vi "Add Channel.vi"(8 "error in (no error)":errorcluster, 11 "Parent Ref in":T3 format="%.0x") -> (0 "error out":errorcluster, 1 "Cancelled?":bool, 2 "Channel Settings":T2, 3 "Parent Ref out":T3 format="%.0x")   [LabVIEW 2011, in "Ethernet IP Custom Device Custom Device.lvlib"]
uses:
  Ethernet IP Custom Device Custom Device.lvlib
  L5K Data Types.ctl
  <vilib>/NI Veristand/Custom Device API/Custom Device Item Ref.ctl
  <vilib>/NI Veristand/Custom Device API/Custom Device API.lvlib
panel:
  in  "Same":bool=TRUE
  in  "Tag Name":string
  in  "Cancel":bool
  in  "OK":bool
  in  "Data Type":T1=enum."REAL"
  in  "Number of Elements":u16=1 min=1 max=256
  in  "Channel Name":string
  # "Please enter the following channel settings:"
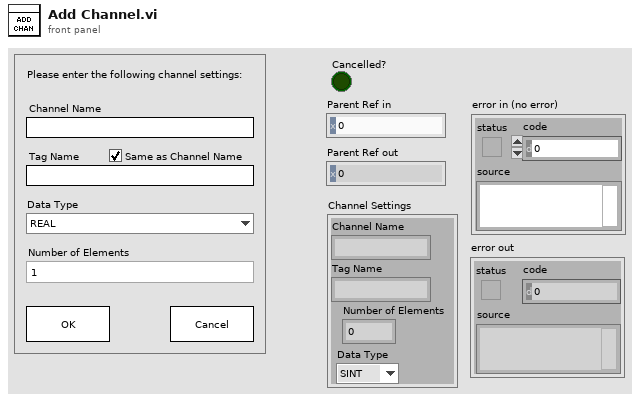
[diagram p1: front panel]
types:
  T1 = typedef "Ethernet IP Custom Device Custom Device.lvlib/L5K Data Types.ctl" = enum16{"SINT", "INT", "DINT", "REAL", "BOOL"}
  T2 = cluster{"Channel Name":string, "Tag Name":string, "Number of Elements":u16, "Data Type":T1}
  T3 = typedef "Custom Device API.lvlib/Custom Device Item Ref.ctl" = u64
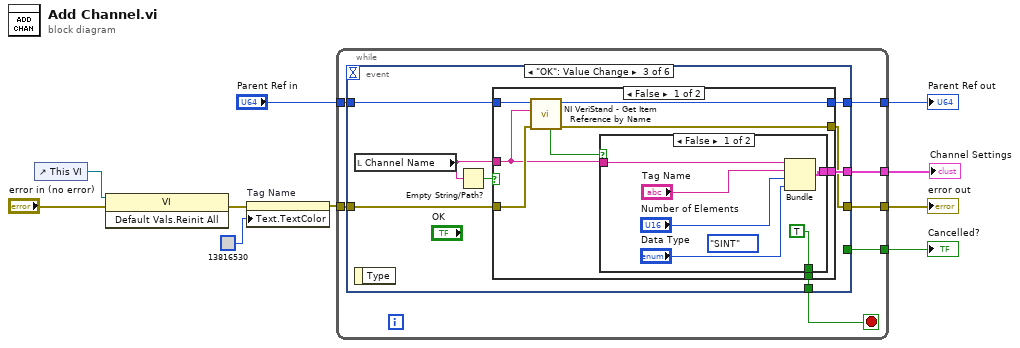
[diagram p0: block diagram]
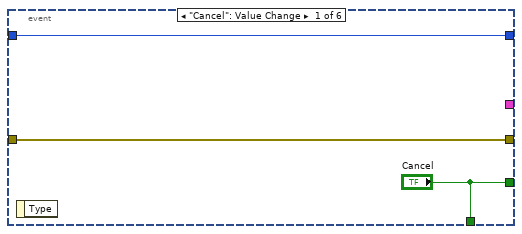
[diagram p2: hidden frame]
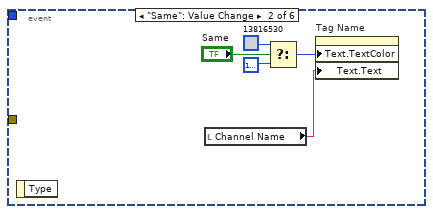
[diagram p3: hidden frame]
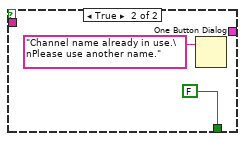
[diagram p4: hidden frame]
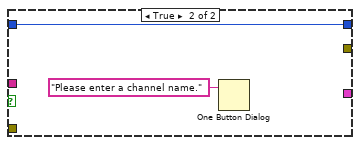
[diagram p5: hidden frame]
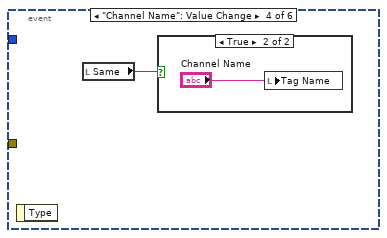
[diagram p6: hidden frame]
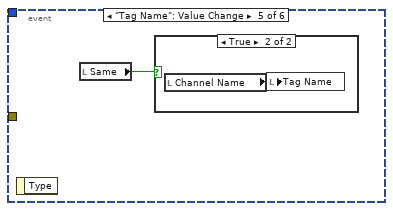
[diagram p8: hidden frame]
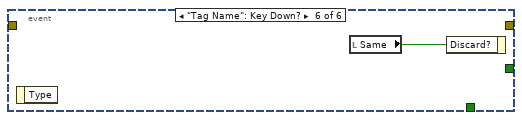
[diagram p10: hidden frame]
diagram:
  n1 = control-ref of="This VI"() -> (w6:refnum<vi>)
  n2 = invoke class="VI" method="Default Vals.Reinit All"(reference=w6, error in="error in (no error)") -> (error out=w4:errorcluster)  [unwired: 1 in, 2 out]
  n3 = property on="Tag Name" class="Str"(error in=w4, "Text.TextColor"=u32 13816530) -> (error out=w3:errorcluster)  [unwired: 1 in, 1 out]
  n4 = while {
    tunnel: "Parent Ref in" -> [w17]
    tunnel: [w15] -> w9
    tunnel: w3 -> [w14]
    tunnel: [w13] -> w1
    tunnel: [w12] -> w8
    tunnel: [w11] -> w7
    stop <- w16 stop-if-true
    n5 = event shown="[2] \"OK\": Value Change" {
      selector: _ -> [_ _ _ _ _ _]
      dyn-events: _ -> [_ _ _ _ _ _]
      timeout: _ -> [_ _ _ _ _ _]
      tunnel: w17 -> [w19 _ w33 _ _ _]
      tunnel: ["Cancel" _ w30 _ _ _] -> w16
      tunnel: ["Cancel" _ _ _ _ _] -> w15
      tunnel: w14 -> [w18 _ w32 _ _ _]
      tunnel: [_ _ w31 _ _ _] -> w13
      tunnel: [w19 _ w29 _ _ _] -> w12
      tunnel: [w18 _ w28 _ _ _] -> w11
      event "Cancel": Value Change {
        n6 = event-data() -> ()  [unwired: 1 in, 1 out]
      }
      event "Same": Value Change {
        n7 = event-data() -> ()  [unwired: 1 in, 1 out]
        n8 = local read "Channel Name"() -> (w22:string)
        n9 = Select(t=u32 13816530, s="Same", f=u32 16777228) -> (s? t:f=w25:u32)
        n10 = property on="Tag Name" class="Str"("Text.TextColor"=w25, "Text.Text"=w22) -> ()  [unwired: 2 in, 2 out]
      }
      event "OK": Value Change {
        n11 = local read "Channel Name"() -> (w26:string)
        n12 = event-data() -> ()  [unwired: 1 in, 1 out]
        n13 = Empty String/Path?(string/path=w26) -> (empty?=w27:bool)
        n14 = case shown="False" w27 {
          tunnel: w33 -> [w41 w50]
          tunnel: w32 -> [w40 _]
          tunnel: w26 -> [w38 _]
          tunnel: [w37 _] -> w31
          tunnel: [w36 _] -> w30
          tunnel: [w35 w50] -> w29
          tunnel: [w34 _] -> w28
          frame False {
            n15 = call <vilib>:"NI VeriStand - Get Item Reference by Name.vi"("error in (no error)"=w40, "Item Name"=w38, "Parent Ref in"=w41) -> ("error out"=w34:errorcluster, "Parent Ref out"=w35:T3, "Found"=w39:bool)  [unwired: 5 in, 1 out]
            n16 = case shown="False" w39 {
              tunnel: w38 -> [w43 _]
              tunnel: [w45 _] -> w37
              tunnel: [TRUE FALSE] -> w36
              frame False {
                (unwired) L5K_Data_Types."SINT" ("Data Type")
                n17 = Bundle("Channel Name"=w43, "Tag Name"="Tag Name", "Number of Elements"="Number of Elements", "Data Type"="Data Type") -> (w45:T2)  [unwired: 1 in]
              }
              frame True {
                n18 = One Button Dialog(message="Channel name already in use.\nPlease use another name.") -> ()  [unwired: 1 in, 1 out]
              }
            }
          }
          frame True {
            n19 = One Button Dialog(message="Please enter a channel name.") -> ()  [unwired: 1 in, 1 out]
          }
        }
      }
      event "Channel Name": Value Change {
        n20 = event-data() -> ()  [unwired: 1 in, 1 out]
        n21 = local read "Same"() -> (w52:bool)
        n22 = case shown="True" w52 {
          frame False {
          }
          frame True {
            n23 = local write "Tag Name"("Channel Name") -> ()
          }
        }
      }
      event "Tag Name": Value Change {
        n24 = event-data() -> ()  [unwired: 1 in, 1 out]
        n25 = local read "Same"() -> (w54:bool)
        n26 = case shown="True" w54 {
          frame False {
          }
          frame True {
            n27 = local read "Channel Name"() -> (w55:string)
            n28 = local write "Tag Name"(w55) -> ()
          }
        }
      }
      event "Tag Name": Key Down? {
        n29 = event-data() -> ()  [unwired: 1 in, 1 out]
        n30 = local read "Same"() -> (w56:bool)
        n31 = event-data("Discard?"=w56) -> ()  [unwired: 1 in, 1 out]
      }
    }
  }
  "Parent Ref out" <- w8
  "Cancelled?" <- w9
  "error out" <- w7
  "Channel Settings" <- w1
